vi "TF_String.vi"(1 "FalseCase":string="False", 2 "Case":bool, 3 "TrueCase":string="True") -> (0 "Result":string)   [LabVIEW 2013]
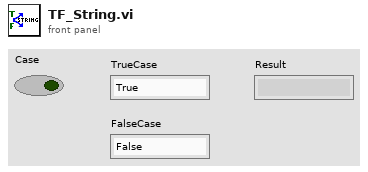
[diagram p1: front panel]
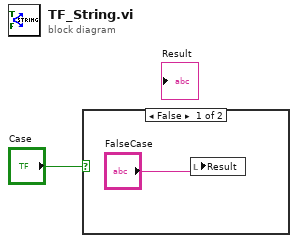
[diagram p0: block diagram]
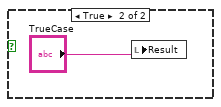
[diagram p2: hidden frame]
diagram:
  n1 = case shown="False" "Case" {
    frame False {
      n2 = local write "Result"("FalseCase") -> ()
    }
    frame True {
      n3 = local write "Result"("TrueCase") -> ()
    }
  }
